vi "DataXML saveXMLProcess.vi"(5 "addTagName":string="System", 7 "dataType":T1, 8 "error in (no error)":errorcluster, 9 "appended path":path, 10 "rootNodeName":string, 11 "newData":string[][](array[string])) -> (0 "error out":errorcluster)   [LabVIEW 2018, in "DataXML.lvclass"]
uses:
  DataXML.lvclass
  DataXML dataType.ctl
  <vilib>/Utility/error.llb/Error Cluster From Error Code.vi
  <vilib>/ErrorRing/Error Ring.xnode
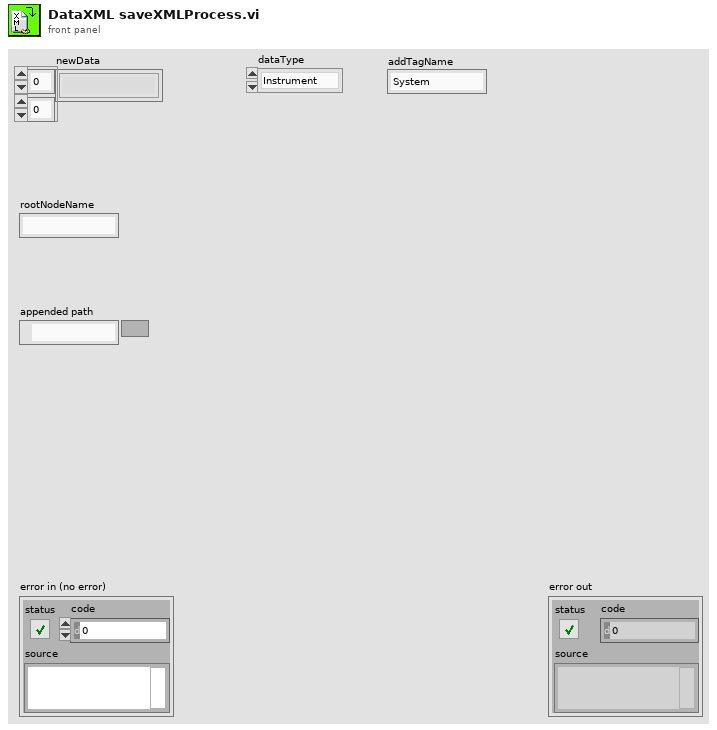
[diagram p1: front panel]
types:
  T1 = typedef "DataXML dataType.ctl" = enum16{"Instrument", "UserInterface", "SampleType", "UserDefined"}
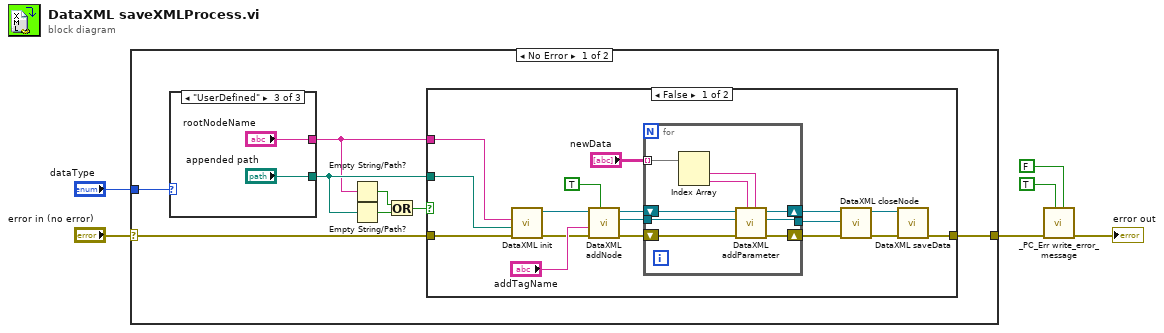
[diagram p0: block diagram]
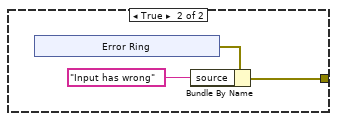
[diagram p2: hidden frame]
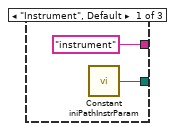
[diagram p3: hidden frame]
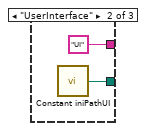
[diagram p4: hidden frame]
diagram:
  n1 = case shown="No Error" "error in (no error)" {
    selector: "error in (no error)" -> [w14 w54]
    tunnel: "dataType" -> [w13 _]
    tunnel: [w12 w54] -> w1
    frame No Error {
      n2 = case shown="\"UserDefined\"" w13 {
        tunnel: [w49 w51 "appended path"] -> w8
        tunnel: ["instrument" ("rootNodeName") "UI" ("rootNodeName") "rootNodeName"] -> w7
        frame "Instrument", Default {
          n3 = call "Constant iniPathInstrParam.vi"() -> ("appended path"=w49:path)
        }
        frame "UserInterface" {
          n4 = call "Constant iniPathUI.vi"() -> ("appended path"=w51:path)
        }
        frame "UserDefined" {
        }
      }
      n5 = Empty String/Path?(string/path=w7) -> (empty?=w11:bool)
      n6 = Empty String/Path?(string/path=w8) -> (empty?=w10:bool)
      n7 = Or(x=w11, y=w10) -> (x .or. y?=w9:bool)
      n8 = case shown="False" w9 {
        tunnel: w14 -> [w31 _]
        tunnel: [w30 w41] -> w12
        tunnel: w8 -> [w15 _]
        tunnel: w7 -> [w16 _]
        frame False {
          n9 = call "DataXML init.vi"("error in (no error)"=w31, "file path"=w15, "root node name"=w16) -> ("error out"=w28:errorcluster, "DataXML out"=w27:refnum<class "DataXML.lvclass">)  [unwired: 7 in]
          n10 = call "DataXML addNode.vi"("add_root? (F)"=TRUE, "error in (no error)"=w28, "add tag name"="addTagName", "DataXML in"=w27) -> ("error out"=w24:errorcluster, "new element"=w23:refnum<k20>, "DataXML out"=w25:refnum<class "DataXML.lvclass">)  [unwired: 5 in]
          n11 = for {
            tunnel: w23 -> [w38]
            shift-right: [w36] -> w20
            shift-left: w24 -> [w39]
            shift-right: [w37] -> w22
            shift-left: w25 -> [w40]
            tunnel: [w35] -> w21
            tunnel: "newData" -> [w34] mode=indexing
            n12 = Index Array(array=w34) -> (element #1=w33:string, element #2=w32:string)  [unwired: 2 in]
            n13 = call "DataXML addParameter.vi"("param name"=w33, "param value"=w32, "error in (no error)"=w39, "tag node in"=w38, "DataXML in"=w40) -> ("error out"=w36:errorcluster, "tag node out"=w35:refnum<k20>, "DataXML out"=w37:refnum<class "DataXML.lvclass">)  [unwired: 4 in]
          }
          n14 = call "DataXML closeNode.vi"("error in (no error)"=w20, "tag node"=w21, "DataXML in"=w22) -> ("error out"=w18:errorcluster, "DataXML out"=w19:refnum<class "DataXML.lvclass">)  [unwired: 7 in]
          n15 = call "DataXML saveData.vi"("error in (no error)"=w18, "DataXML in"=w19) -> ("error out"=w30:errorcluster)  [unwired: 8 in, 1 out]
        }
        frame True {
          n16 = xnode "Error Ring"() -> ("error out"=w43:errorcluster)
          n17 = Bundle By Name(cluster=w43, "source"="Input has wrong") -> (w41:errorcluster)
        }
      }
    }
    frame Error {
    }
  }
  n18 = call "_PC_Err write_error_message.vi"("skipWrong( T )"=FALSE ("skipWrong"), "show msg( T )"=TRUE, "error in"=w1) -> ("error out"=→"error out":errorcluster)  [unwired: 8 in]
